vi "Get settings chain.vi"(8 "error in (no error)":errorcluster, 11 "AOTFBase in":refnum<class "AOTF.lvclass">) -> (0 "error out":errorcluster, 1 "class name":string[](array[string]), 2 "settings":variant[](array[variant]), 3 "AOTFBase out":refnum<class "AOTF.lvclass">)   [LabVIEW 2012, in "AOTF.lvclass"]
doc: "Returns an array of variants containing the settings clusters of each class in the inheritance chain (lowest child class first), together with an array of all class names in the inheritance chain.\n\nFor classes without settings cluster, the settings chain contains empty variants."
uses:
  AOTF.lvclass
  <vilib>/Distrio/Murmex/Murmex/Murmex.lvclass
  AOTF.lvclass/AOTF.ctl
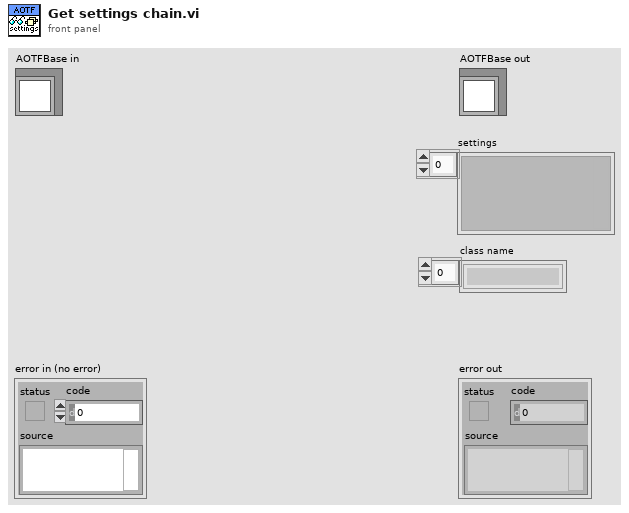
[diagram p1: front panel]
types:
  T1 = typedef "AOTF.lvclass/Settings cluster.ctl" = cluster{"Wavelength":T2, "Power":dbl}
  T2 = typedef "AOTF.lvclass/laser line ring.ctl" = u8
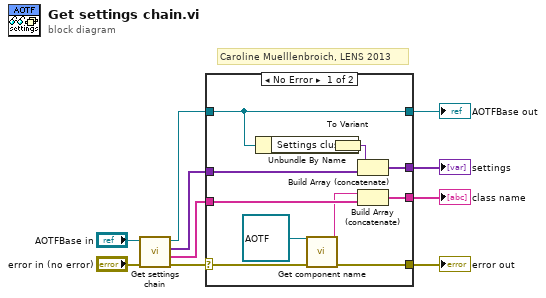
[diagram p0: block diagram]
diagram:
  # "Caroline Muelllenbroich, LENS 2013"
  n1 = call-parent "Get settings chain.vi"("error in (no error)"="error in (no error)", "MurmexBase in"="AOTFBase in") -> ("error out"=w8:errorcluster, "class name"=w4:string[], "settings"=w7:variant[], "MurmexBase out"=w1:refnum<class "AOTF.lvclass">)  [unwired: 6 in]
  n2 = case shown="No Error" w8 {
    selector: w8 -> [w21 w25]
    tunnel: w7 -> [w17 w23]
    tunnel: w1 -> [w16 w22]
    tunnel: [w16 w22] -> w5
    tunnel: [w15 w23] -> w6
    tunnel: w4 -> [w14 w24]
    tunnel: [w12 w24] -> w3
    tunnel: [w11 w25] -> w2
    frame No Error {
      n3 = Unbundle By Name(w16) -> ("Settings cluster"=w19:T1)
      n4 = call <vilib>:"Get component name.vi"("error in (no error)"=w21, "Murmex in"=refnum<class "AOTF.lvclass"> refnum ("AOTF")) -> ("error out"=w11:errorcluster, "component name"=w13:string)  [unwired: 7 in, 1 out]
      n5 = To Variant(anything=w19) -> (Variant=w18:variant)
      n6 = Build Array (concatenate)(w18, w17) -> (w15:variant[])
      n7 = Build Array (concatenate)(w13, w14) -> (w12:string[])
    }
    frame Error {
    }
  }
  "error out" <- w2
  "AOTFBase out" <- w5
  "settings" <- w6
  "class name" <- w3
